vi "subVI_STS_ramp.vi"(8 "Ramp Vpp":dbl=3.0, 9 "Ramp offset":dbl, 10 "Ramp datapoints":i16=5000, 11 "n":i64) -> (2 "n1":dbl, 3 "Ramp out":dbl)   [LabVIEW 2019]
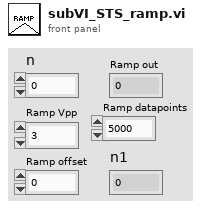
[diagram p1: front panel]
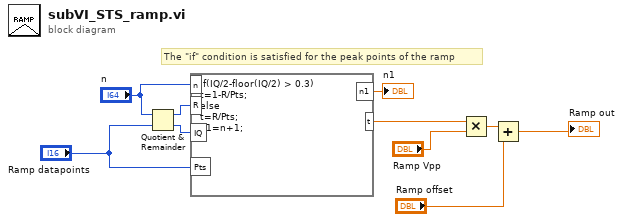
[diagram p0: block diagram]
diagram:
  # "The \"if\" condition is satisfied for the peak points of the ramp"
  n1 = Quotient & Remainder(x="n", y="Ramp datapoints") -> (x-y*floor(x/y)=w9:i64, floor(x/y)=w8:i64)
  n2 = formula code="if(IQ/2-floor(IQ/2) > 0.3)\nt=1-R/Pts;\nelse\nt=R/Pts;\nn1=n+1;"("R"=w9, "IQ"=w8, "Pts"="Ramp datapoints", "n"="n") -> ("t"=w10:dbl, "n1"=→"n1":dbl)
  n3 = Multiply(x=w10, y="Ramp Vpp") -> (x*y=w5:dbl)
  n4 = Add(x=w5, y="Ramp offset") -> (x+y=→"Ramp out":dbl)
